vi "CheckDataUsingChecksum.vi"(11 "hex in":string="\bU\u0004\u0000\u0000\u0000\u0001\u0000b") -> (1 "x = y?":bool, 2 "checksum value":string, 3 "hex out":string)   [LabVIEW 2018]
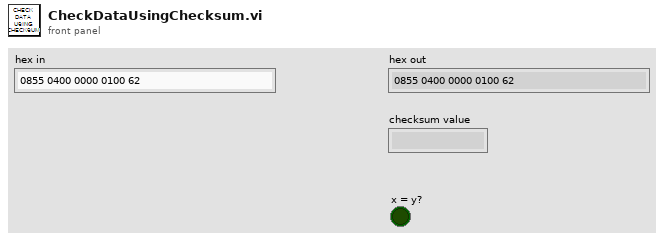
[diagram p1: front panel]
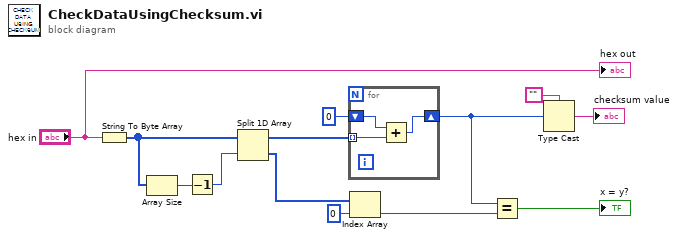
[diagram p0: block diagram]
diagram:
  n1 = String To Byte Array(string="hex in") -> (unsigned byte array=w12:u8[])
  n2 = Array Size(array=w12) -> (size(s)=w13:i32)
  n3 = Decrement(x=w13) -> (x-1=w11:i32)
  n4 = Split 1D Array(array=w12, index=w11) -> (first subarray=w9:u8[], second subarray=w6:u8[])
  n5 = for {
    tunnel: w9 -> [w16] mode=indexing
    shift-right: [w14] -> w3
    shift-left: u8 0 -> [w15]
    n6 = Add(x=w15, y=w16) -> (x+y=w14:u8)
  }
  n7 = Index Array(array=w6, index=0 ("인덱스")) -> (element=w4:u8)
  n8 = Equal?(x=w3, y=w4) -> (x = y?=→"x = y?":bool)
  n9 = Type Cast(type="", x=w3) -> (*(type *) &x=→"checksum value":string)
  "hex out" <- "hex in"
